vi "emi_Set Window header text.vi"(5 "VI Refnum(This VI)":refnum<vi>, 7 "Header String":string, 9 "error in (no error)":errorcluster, 13 "Use Version info(F)":bool) -> (6 "VI Refnum":refnum<vi>, 10 "error out":errorcluster)   [LabVIEW 2011]
doc: "Set VI FP Header tittle. If selected, and version information available, this is used in header\n\nOn Error: No Action"
uses:
  0 - General/App/Version/Private/_emi_Version Holder.vi
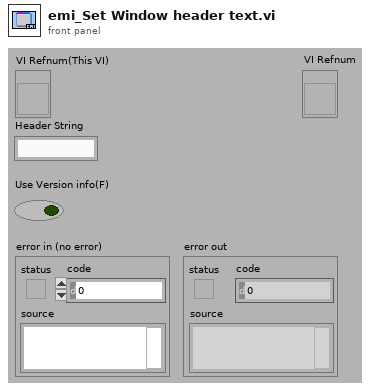
[diagram p1: front panel]
types:
  T1 = typedef "emi_Version Info.ctl" = cluster{"Name":string, "Major":i16, "Minor":i16, "Fix":i16, "Build":i32, "Type":enum16{"Alfa", "Beta", "Stable"}, "Dev":bool, "Version Name":string, "Date":timestamp}
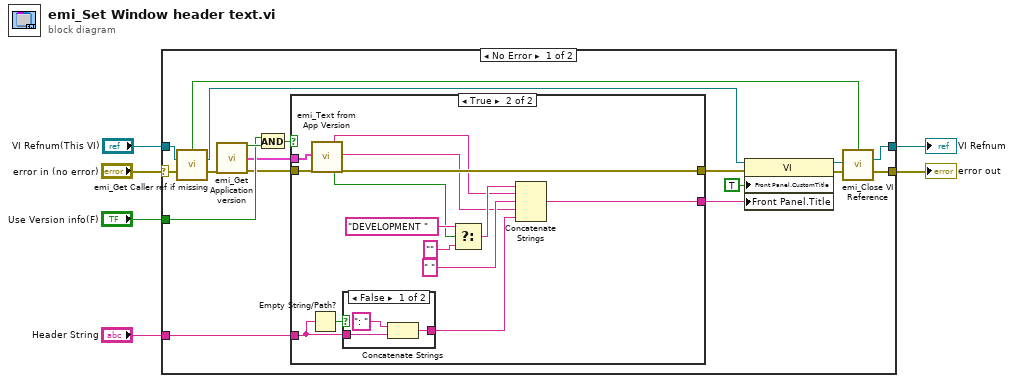
[diagram p0: block diagram]
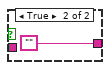
[diagram p3: hidden frame]
diagram:
  n1 = case shown="No Error" "error in (no error)" {
    selector: "error in (no error)" -> [w22 w45]
    tunnel: "VI Refnum(This VI)" -> [w18 w46]
    tunnel: [w19 w46] -> w5
    tunnel: [w20 w45] -> w4
    tunnel: "Header String" -> [w7 _]
    tunnel: "Use Version info(F)" -> [w12 _]
    frame No Error {
      n2 = call "emi_Get Caller ref if missing.vi"("VI Refnum(Calling VI)"=w18, "error in (no error)"=w22) -> ("Ref Generated"=w23:bool, "VI Refnum Out"=w16:refnum<vi>, "error out"=w15:errorcluster)  [unwired: 11 in]
      n3 = call "emi_Get Application version.vi"("error in (no error)"=w15) -> ("Version has been set"=w13:bool, "Version Info out"=w9:T1, "error out"=w10:errorcluster)  [unwired: 12 in]
      n4 = And(x=w12, y=w13) -> (x .and. y?=w11:bool)
      n5 = case shown="True" w11 {
        tunnel: w10 -> [w26 w40]
        tunnel: [w26 w39] -> w14
        tunnel: w9 -> [_ w38]
        tunnel: [w25 w27] -> w8
        tunnel: w7 -> [w25 w36]
        frame False {
        }
        frame True {
          n6 = Empty String/Path?(string/path=w36) -> (empty?=w37:bool)
          n7 = call "emi_Text from App Version.vi"("Version Info"=w38, "error in (no error)"=w40) -> ("Name"=w29:string, "Dev Only Version"=w31:bool, "Short version Type"=w30:string, "error out"=w39:errorcluster)  [unwired: 8 in, 6 out]
          n8 = case shown="False" w37 {
            tunnel: w36 -> [w41 _]
            tunnel: [w43 ""] -> w28
            frame False {
              n9 = Concatenate Strings(": ", w41) -> (w43:string)
            }
            frame True {
            }
          }
          n10 = Select(t="DEVELOPMENT " ("Version Short"), s=w31, f="") -> (s? t:f=w32:string)
          n11 = Concatenate Strings(w32, w29, " " ("string"), w30, w28) -> (w27:string)
        }
      }
      n12 = property class="VI"(reference=w16, error in=w14, "Front Panel.CustomTitle"=TRUE ("Front Panel Window:Custom Title"), "Front Panel.Title"=w8) -> (reference out=w17:refnum<vi>, error out=w21:errorcluster)
      n13 = call "emi_Close VI Reference.vi"("Close ref?(T)"=w23, "VI Refnum"=w17, "error in (no error)"=w21) -> ("VI Refnum Out"=w19:refnum<vi>, "error out"=w20:errorcluster)  [unwired: 11 in]
    }
    frame Error {
    }
  }
  "error out" <- w4
  "VI Refnum" <- w5
